vi "Stop Pump.vi"(0 "reference in":refnum<class "Stand.lvclass">, 11 "error in (no error)":errorcluster) -> (4 "reference out":refnum<class "Stand.lvclass">, 6 "Done":bool, 15 "error out":errorcluster)   [LabVIEW 2019, in "Stand.lvclass"]
uses:
  Stand.lvclass
  C:/Users/ANENKOV_V1/Desktop/src/Device_class/Device.lvclass
  FPGA/TypeDef/DO index.ctl
  Device_class/Device.lvclass/Device.ctl
  Stand.lvclass/Stand.ctl
  TypeDef/Active Motor.ctl
  TypeDef/Motor N.ctl
  FPGA_API_class/FPGA API.lvclass
  Device_class/Device.lvclass
  PM_Group_class/PM_Group.lvclass
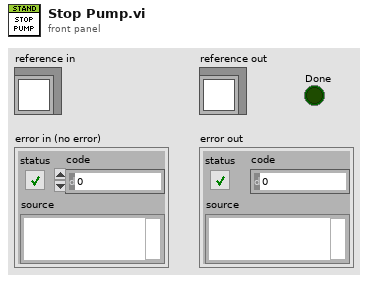
[diagram p1: front panel]
types:
  T1 = typedef "DO index.ctl" = u8
  T2 = typedef "Active Motor.ctl" = cluster{"Active":bool, "MotorN":T3}
  T3 = typedef "Motor N.ctl" = enum16{"M12", "M21", "M24"}
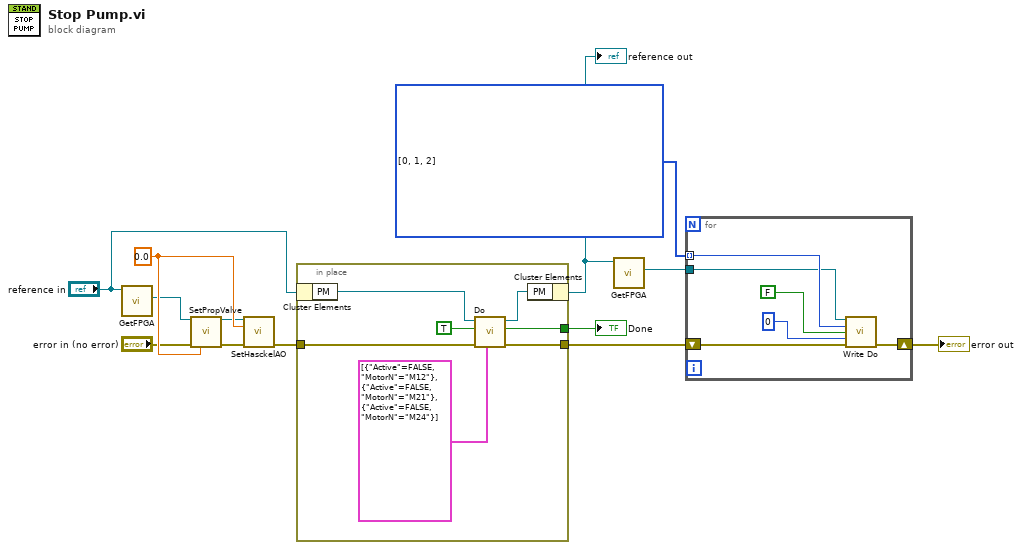
[diagram p0: block diagram]
diagram:
  w1 = T1[] [0, 1, 2] items=["DO 0 [KP1 [DO 0]]", "DO 1 [ON KP2 [DO 1]]", "DO 2 [ON KP3 [DO 2]]", "DO 3 [WATER Y18.1 [DO3]]", "DO 4 [WATER Y18.2 [DO4]]", "DO 5 [KP6 Y29.1 33.7]", "DO 6 [KP7 Y29.2 33.8]", "DO 7 [KP8 Y29.3 33.9]", "DO 8 [KP9 Y29.4  33.12]", "DO 9 [KP10 Y29.5 33.1]", "DO 10 [KP11 Y29.6 33.2]", "DO 11 [KP12 Y29.7  33.13]", "DO 12 [KP13 Y29.8  33.11]", "DO 13 [KP14 Y29.9 33.10]", "DO 14 [KP15 Y29.10  33.6]", "DO 15 [KP16 Y29.11  33.5]", "DO 16 [KP17 Y29.12  33.4]", "DO 17 [KP18 Y29.13 33.3]", "DO 18 [AIR KP19]", "DO 19 [STEP DRIVE EN KP20]", "DO 20 [KP21 Y44.1 OPEN]", "DO 21 [ KP22 Y44.1 CLOSE]", "DO 22 [ KP23 Y44.2 OPEN]", "DO 23", "DO 24 [STEP DRIVE 1]", "DO 25 [STEP DRIVE 2]"]
  w13 = 0.0 ("AO 1")
  n1 = call "GetFPGA.vi"("Device in"="reference in") -> ("FPGA API.lvclass"=w9:refnum<class "FPGA API.lvclass">)  [unwired: 10 in]
  n2 = call-dynamic "SetPropValve.vi"("FPGA API in"=w9, "error in (no error)"="error in (no error)", "AO 1"=w13) -> ("FPGA API out"=w10:refnum<class "FPGA API.lvclass">, "error out"=w11:errorcluster)  [unwired: 11 in]
  n3 = call-dynamic "SetHasckelAO.vi"("FPGA API in"=w10, "Haskel in"=w13, "error in (no error)"=w11) -> ("error out"=w12:errorcluster)  [unwired: 11 in, 1 out]
  n4 = in-place {
    in-place-border: w12 -> [w19]
    in-place-border: [w17] -> w3
    in-place-border: [w14] -> w6
    n5 = in-place-cluster #1("reference in") -> ("PM"=w20:refnum<class "PM_Group.lvclass">)
    n6 = call "Do.vi"("Data"=T2[] [{"Active"=FALSE, "MotorN"=enum."M12"}, {"Active"=FALSE, "MotorN"=enum."M21"}, {"Active"=FALSE, "MotorN"=enum."M24"}] ("Array"), "error in (no error)"=w19, "Do"=TRUE, "PM_Group in"=w20) -> ("error out"=w17:errorcluster, "Done"=w14:bool, "PM_Group out"=w18:refnum<class "PM_Group.lvclass">)  [unwired: 5 in]
    n7 = in-place-cluster #1("PM"=w18) -> (w4:refnum<class "Stand.lvclass">)
  }
  "reference out" <- w4
  "Done" <- w6
  n8 = call "GetFPGA.vi"("Device in"=w4) -> ("FPGA API.lvclass"=w5:refnum<class "FPGA API.lvclass">)  [unwired: 10 in]
  n9 = for {
    tunnel: w1 -> [w26] mode=indexing
    tunnel: w5 -> [w23]
    shift-right: [w21] -> w2
    shift-left: w3 -> [w22]
    n10 = call-dynamic "Write Do.vi"("FPGA API in"=w23, "#DO"=w26, "value"=FALSE, "Time uSec"=u32 0, "error in (no error)"=w22) -> ("error out"=w21:errorcluster)  [unwired: 9 in, 1 out]
  }
  "error out" <- w2
